vi "BASE.Device.GetConfig.vi"(8 "error in (no error)":errorcluster, 11 "BASE.Device in":refnum<class "BASE.Device.lvclass">) -> (0 "error out":errorcluster, 2 "config":T1, 3 "BASE.Device out":refnum<class "BASE.Device.lvclass">)   [LabVIEW 2019, in "BASE.Device.lvlib" / "BASE.Device.lvclass"]
uses:
  BASE.Device.lvclass
  config--cluster.ctl
  BASE.Device.lvclass/BASE.Device.ctl
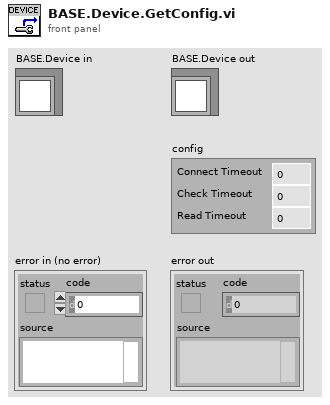
[diagram p1: front panel]
types:
  T1 = typedef "BASE.Device.lvlib/BASE.Device.lvclass/config--cluster.ctl" = cluster{"Connect Timeout":i32, "Check Timeout":i32, "Read Timeout":i32}
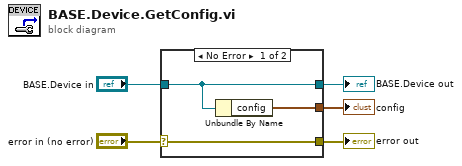
[diagram p0: block diagram]
diagram:
  n1 = case shown="No Error" "error in (no error)" {
    selector: "error in (no error)" -> [w8 w9]
    tunnel: [w8 w9] -> w4
    tunnel: [w7 w10] -> w2
    tunnel: "BASE.Device in" -> [w7 w10]
    tunnel: [w6 _] -> w1
    frame No Error {
      n2 = Unbundle By Name(w7) -> ("config"=w6:T1)
    }
    frame Error {
    }
  }
  "error out" <- w4
  "BASE.Device out" <- w2
  "config" <- w1
